vi "ReadPixelU64.vi"(8 "error in":errorcluster, 9 "Y Coordinate":i32, 10 "X Coordinate":i32, 11 "Image Reference In":T1) -> (0 "error out":errorcluster, 2 "Pixel value":u64, 3 "Image Reference Out":T1)   [LabVIEW 2020, in "OpenLvVision_Image.lvlib" / "DataAccess.lvlib"]
doc: "Provides the pixel's value at the given coordinates."
uses:
  DataAccess.lvlib
  Management/TypeDef/Image.ctl
  <vilib>/Utility/error.llb/Error Cluster From Error Code.vi
  <vilib>/ErrorRing/Error Ring.xnode
  Management/Management.lvlib
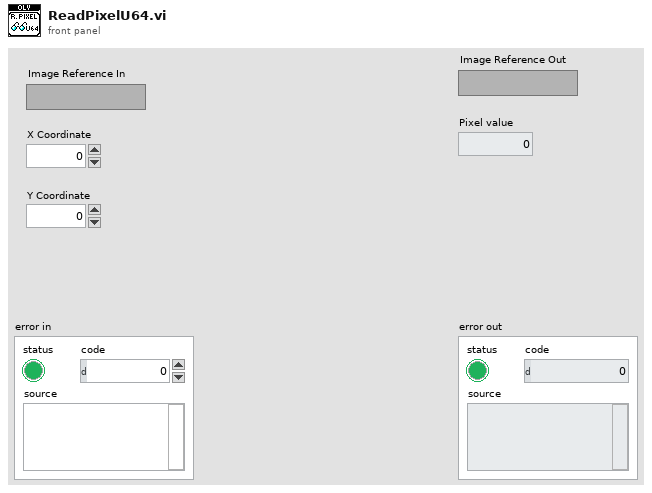
[diagram p1: front panel]
types:
  T1 = typedef "OpenLvVision_Image.lvlib/Management.lvlib/Image.ctl" = refnum<image>
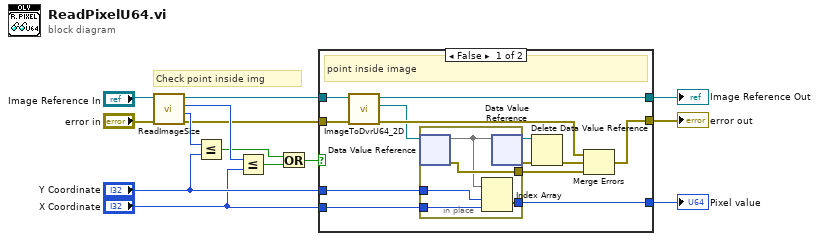
[diagram p0: block diagram]
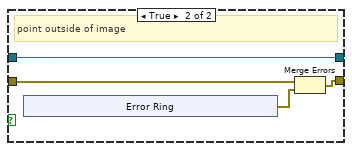
[diagram p2: hidden frame]
diagram:
  # "Check point inside img"
  n1 = call "ReadImageSize.vi"("error in"="error in", "Image Reference In"="Image Reference In") -> ("error out"=w4:errorcluster, "Height"=w10:i32, "Width"=w12:i32, "Image Reference Out"=w11:T1)  [unwired: 6 in]
  n2 = Less Or Equal?(x=w10, y="Y Coordinate") -> (x <= y?=w8:bool)
  n3 = Less Or Equal?(x=w12, y="X Coordinate") -> (x <= y?=w9:bool)
  n4 = Or(x=w8, y=w9) -> (x .or. y?=w7:bool)
  n5 = case shown="False" w7 {
    tunnel: w11 -> [w27 w34]
    tunnel: w4 -> [w26 w36]
    tunnel: "Y Coordinate" -> [w18 _]
    tunnel: "X Coordinate" -> [w17 _]
    tunnel: [w25 w34] -> w3
    tunnel: [w15 w33] -> w2
    tunnel: [w16 _] -> w1
    frame False {
      # "point inside image"
      n6 = call "ImageToDvrU64_2D.vi"("error in"=w26, "Image Reference In"=w27) -> ("error out"=w20:errorcluster, "EDVR 2D U64"=w19:refnum<data-value>, "Image Reference Out"=w25:T1)  [unwired: 6 in, 1 out]
      n7 = in-place {
        in-place-border: [w32] -> w23
        in-place-border: w18 -> [w30]
        in-place-border: w17 -> [w29]
        in-place-border: [w28] -> w16
        n8 = in-place-dvr #1(w19) -> (w31:u64[][], w32:errorcluster)
        n9 = Index Array(array=w31, index (row)=w30, index (col)=w29) -> (element=w28:u64)
        n10 = in-place-dvr #1(w31) -> (w21:refnum<data-value>, w22:errorcluster)
      }
      n11 = Delete Data Value Reference(data value reference=w21, error in=w22) -> (error out=w24:errorcluster)  [unwired: 1 out]
      n12 = Merge Errors(w20, w24, w23) -> (w15:errorcluster)
    }
    frame True {
      # "point outside of image"
      n13 = xnode "Error Ring"() -> ("error out"=w35:errorcluster)
      n14 = Merge Errors(w36, w35) -> (w33:errorcluster)
    }
  }
  "error out" <- w2
  "Image Reference Out" <- w3
  "Pixel value" <- w1
